vi "Flatten.vi"(11 "Data Out in":dbl[][][](array[numeric])) -> (3 "Data Out out":dbl[](array[numeric]))   [LabVIEW 2015]
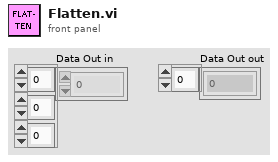
[diagram p1: front panel]
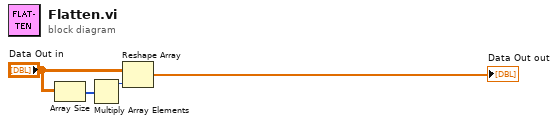
[diagram p0: block diagram]
diagram:
  n1 = Array Size(array="Data Out in") -> (size(s)=w1:i32[])
  n2 = Multiply Array Elements(1:w1) -> (0:w2:i32)
  n3 = Reshape Array("Data Out in", w2) -> (→"Data Out out":dbl[])
